vi "PH_Sound.Voegel 2.vi"() -> (0 "... alle Vögel, alle.":cluster{"Tone":dbl, "Beats":i32}[](array[cluster]))   [LabVIEW 2009, in "PH_Sound.lvlib"]
doc: "\"... alle Voegel, alle!."
uses:
  PH_Sound.lvlib
  PH_Common/PH_Audio/PH_3Oktaves.ctl
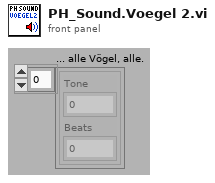
[diagram p1: front panel]
types:
  T1 = typedef "PH_3Oktaves.ctl" = dbl
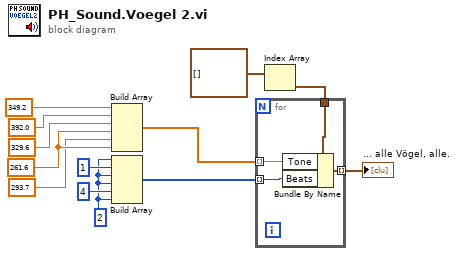
[diagram p0: block diagram]
diagram:
  w4 = u32 2 ("y")
  w11 = T1 293.7 items=["c"=130.8, "cis"=138.6, "d"=146.8, "es"=155.6, "e"=164.8, "f"=174.6, "fis"=185.0, "g"=196.0, "as"=207.6, "a"=220.0, "b"=233.1, "h"=246.9, "c'"=261.6, "cis'"=277.2, "d'"=293.7, "es'"=311.1, "e'"=329.6, "f'"=349.2, "fis'"=370.0, "g'"=392.0, "as'"=415.3, "a'"=440.0, "b'"=466.2, "h'"=493.9, "c''"=523.3, "cis''"=554.4, "d''"=587.3, "es''"=622.3, "e''"=659.3, "f''"=689.5, "fis''"=740.0, "g''"=784.0, "as''"=830.6, "a''"=880.0, "b''"=932.3, "h''"=987.8, "c'''"=1047.0] ("3 Octaves")
  w13 = T1 261.6 items=["c"=130.8, "cis"=138.6, "d"=146.8, "es"=155.6, "e"=164.8, "f"=174.6, "fis"=185.0, "g"=196.0, "as"=207.6, "a"=220.0, "b"=233.1, "h"=246.9, "c'"=261.6, "cis'"=277.2, "d'"=293.7, "es'"=311.1, "e'"=329.6, "f'"=349.2, "fis'"=370.0, "g'"=392.0, "as'"=415.3, "a'"=440.0, "b'"=466.2, "h'"=493.9, "c''"=523.3, "cis''"=554.4, "d''"=587.3, "es''"=622.3, "e''"=659.3, "f''"=689.5, "fis''"=740.0, "g''"=784.0, "as''"=830.6, "a''"=880.0, "b''"=932.3, "h''"=987.8, "c'''"=1047.0] ("3 Octaves")
  w12 = T1 329.6 items=["c"=130.8, "cis"=138.6, "d"=146.8, "es"=155.6, "e"=164.8, "f"=174.6, "fis"=185.0, "g"=196.0, "as"=207.6, "a"=220.0, "b"=233.1, "h"=246.9, "c'"=261.6, "cis'"=277.2, "d'"=293.7, "es'"=311.1, "e'"=329.6, "f'"=349.2, "fis'"=370.0, "g'"=392.0, "as'"=415.3, "a'"=440.0, "b'"=466.2, "h'"=493.9, "c''"=523.3, "cis''"=554.4, "d''"=587.3, "es''"=622.3, "e''"=659.3, "f''"=689.5, "fis''"=740.0, "g''"=784.0, "as''"=830.6, "a''"=880.0, "b''"=932.3, "h''"=987.8, "c'''"=1047.0] ("3 Octaves")
  w9 = T1 392.0 items=["c"=130.8, "cis"=138.6, "d"=146.8, "es"=155.6, "e"=164.8, "f"=174.6, "fis"=185.0, "g"=196.0, "as"=207.6, "a"=220.0, "b"=233.1, "h"=246.9, "c'"=261.6, "cis'"=277.2, "d'"=293.7, "es'"=311.1, "e'"=329.6, "f'"=349.2, "fis'"=370.0, "g'"=392.0, "as'"=415.3, "a'"=440.0, "b'"=466.2, "h'"=493.9, "c''"=523.3, "cis''"=554.4, "d''"=587.3, "es''"=622.3, "e''"=659.3, "f''"=689.5, "fis''"=740.0, "g''"=784.0, "as''"=830.6, "a''"=880.0, "b''"=932.3, "h''"=987.8, "c'''"=1047.0] ("3 Octaves")
  w10 = T1 349.2 items=["c"=130.8, "cis"=138.6, "d"=146.8, "es"=155.6, "e"=164.8, "f"=174.6, "fis"=185.0, "g"=196.0, "as"=207.6, "a"=220.0, "b"=233.1, "h"=246.9, "c'"=261.6, "cis'"=277.2, "d'"=293.7, "es'"=311.1, "e'"=329.6, "f'"=349.2, "fis'"=370.0, "g'"=392.0, "as'"=415.3, "a'"=440.0, "b'"=466.2, "h'"=493.9, "c''"=523.3, "cis''"=554.4, "d''"=587.3, "es''"=622.3, "e''"=659.3, "f''"=689.5, "fis''"=740.0, "g''"=784.0, "as''"=830.6, "a''"=880.0, "b''"=932.3, "h''"=987.8, "c'''"=1047.0] ("3 Octaves")
  n1 = Build Array(w10, w9, w12, w13, w11, w13) -> (w7:T1[])
  n2 = Build Array(w4, 1 ("length"), w4, w4, u32 4 ("y"), w4) -> (w3:u32[])
  n3 = Index Array(array=cluster{"Tone":dbl, "Beats":i32}[] [] ("Song")) -> (element=w1:cluster{"Tone":dbl, "Beats":i32})  [unwired: 1 in]
  n4 = for {
    tunnel: w7 -> [w16] mode=indexing
    tunnel: w1 -> [w17]
    tunnel: [w15] -> w8 mode=indexing
    tunnel: w3 -> [w14] mode=indexing
    n5 = Bundle By Name(cluster=w17, "Tone"=w16, "Beats"=w14) -> (w15:cluster{"Tone":dbl, "Beats":i32})
  }
  "... alle Vögel, alle." <- w8
